vi "Configure Multi Eval Meas Trigger Timeout.vi"(7 "Measurement Trigger Timeout (0.1)":dbl=0.1 format="%^.3e", 8 "error in (no error)":errorcluster, 9 "Trigger Timeout Enabled (Off)":bool, 10 "Instance (1)":T1=1, 11 "VISA resource name":refnum<visa-resource-name>) -> (0 "error out":errorcluster, 3 "VISA resource name out":refnum<visa-resource-name>)   [LabVIEW 2020, in "Rohde&Schwarz CMXP NR FR2 Measurement.lvlib"]
doc: "Selects the maximum time that the measurement waits for a trigger event before it stops in remote control mode or indicates a trigger timeout in manual operation mode. This setting has no influence on 'Free Run' measurements.\n\nAttributes:\nRSCMXPNRFR2M_ATTR_MULTI_EVAL_MEASUREMENT_TRIGGER_TIMEOUT\nRSCMXPNRFR2M_ATTR_MULTI_EVAL_MEASUREMENT_TRIGGER_TIMEOUT_ENABLED\n\nRemote-control command:\nTRIGger:NRMMw:MEAS<i>:MEValuation:TOUT"
uses:
  <instrlib>/Rohde&Schwarz CMXP NR FR2 Measurement/Rohde&Schwarz CMXP NR FR2 Measurement.lvlib
  <instrlib>/Rohde&Schwarz CMXP NR FR2 Measurement/Private/_Instance.ctl
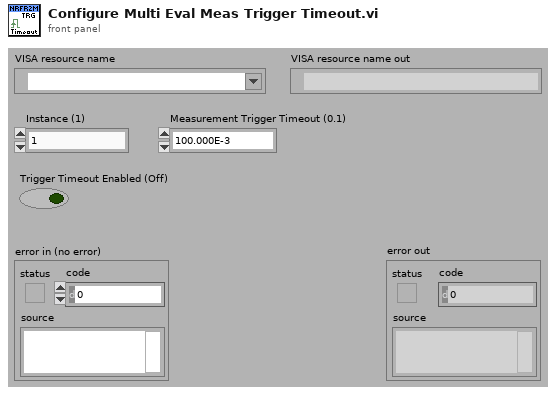
[diagram p1: front panel]
types:
  T1 = typedef "Rohde&Schwarz CMXP NR FR2 Measurement.lvlib/_Instance.ctl" = i32
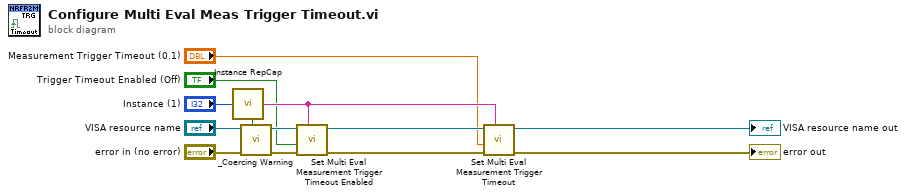
[diagram p0: block diagram]
diagram:
  n1 = call <instrlib>:"Instance RepCap.vi"("Instance In"="Instance (1)") -> ("In Range?"=w7:bool, "RepCap Identifier Out"=w6:string)  [unwired: 1 in]
  n2 = call <instrlib>:"_Coercing Warning.vi"("In Range?"=w7, "error in (no error)"="error in (no error)", "VISA resource name"="VISA resource name") -> ("error out"=w4:errorcluster, "VISA resource name out"=w5:refnum<visa-resource-name>)  [unwired: 7 in]
  n3 = call "Set Multi Eval Measurement Trigger Timeout Enabled"("Repeated Capabilities"=w6, "error in (no error)"=w4, "Multi Eval Measurement Trigger Timeout Enabled (OFF)"="Trigger Timeout Enabled (Off)", "instrument handle"=w5) -> ("error out"=w10:errorcluster, "instrument handle out"=w11:refnum<visa-resource-name>)  [unwired: 6 in]
  n4 = call "Set Multi Eval Measurement Trigger Timeout"("Repeated Capabilities"=w6, "error in (no error)"=w10, "Multi Eval Measurement Trigger Timeout (0.0)"="Measurement Trigger Timeout (0.1)", "instrument handle"=w11) -> ("error out"=→"error out":errorcluster, "instrument handle out"=→"VISA resource name out":refnum<visa-resource-name>)  [unwired: 6 in]
